vi "low_pass_filter_1st.vi"(7 "Input":dbl format="%.2f", 13 "Corner period":dbl(slide)=10.237739663395852 scale=1.0..1000.0) -> (8 "Output":dbl format="%.2f")   [LabVIEW 2016]
doc: "Use this VI to filter a signal using 1st order low pass filter. The difference equation is \nVo(j) = [bVi(j) +Vo(j-1)]/[b+1].\n\nInputs:\nInput,\nCorner period.\nOutputs:\nOutput.\n\nMuhannad Alghamdi\nCSUSB Physics 350"
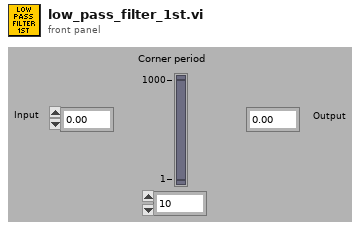
[diagram p1: front panel]
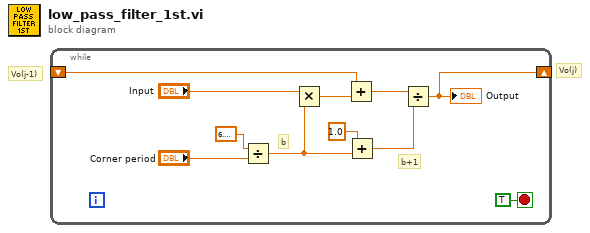
[diagram p0: block diagram]
diagram:
  # "Vo(j-1)"
  # "Vo(j)"
  n1 = while {
    shift-left: _ -> [w1]
    shift-right: [w3] -> _
    stop <- TRUE stop-if-true
    # "b+1"
    # "b"
    n2 = Divide(x=6.283185307179586, y="Corner period") -> (x/y=w6:dbl)
    n3 = Multiply(x="Input", y=w6) -> (x*y=w2:dbl)
    n4 = Add(x=w1, y=w2) -> (x+y=w5:dbl)
    n5 = Add(x=1.0, y=w6) -> (x+y=w4:dbl)
    n6 = Divide(x=w5, y=w4) -> (x/y=w3:dbl)
    "Output" <- w3
  }
